vi "2.2.vi"() -> ()   [LabVIEW 2020]
panel:
  out "Valor\nMinimo":dbl
  out "Valor\nMaximo":dbl
  out "Resultados":dbl[][](array[numeric])
  out "Grafica":dbl[](graph)
  # "Grados \nCelsius"
  # "Fahrenheit"
  # "EMA"
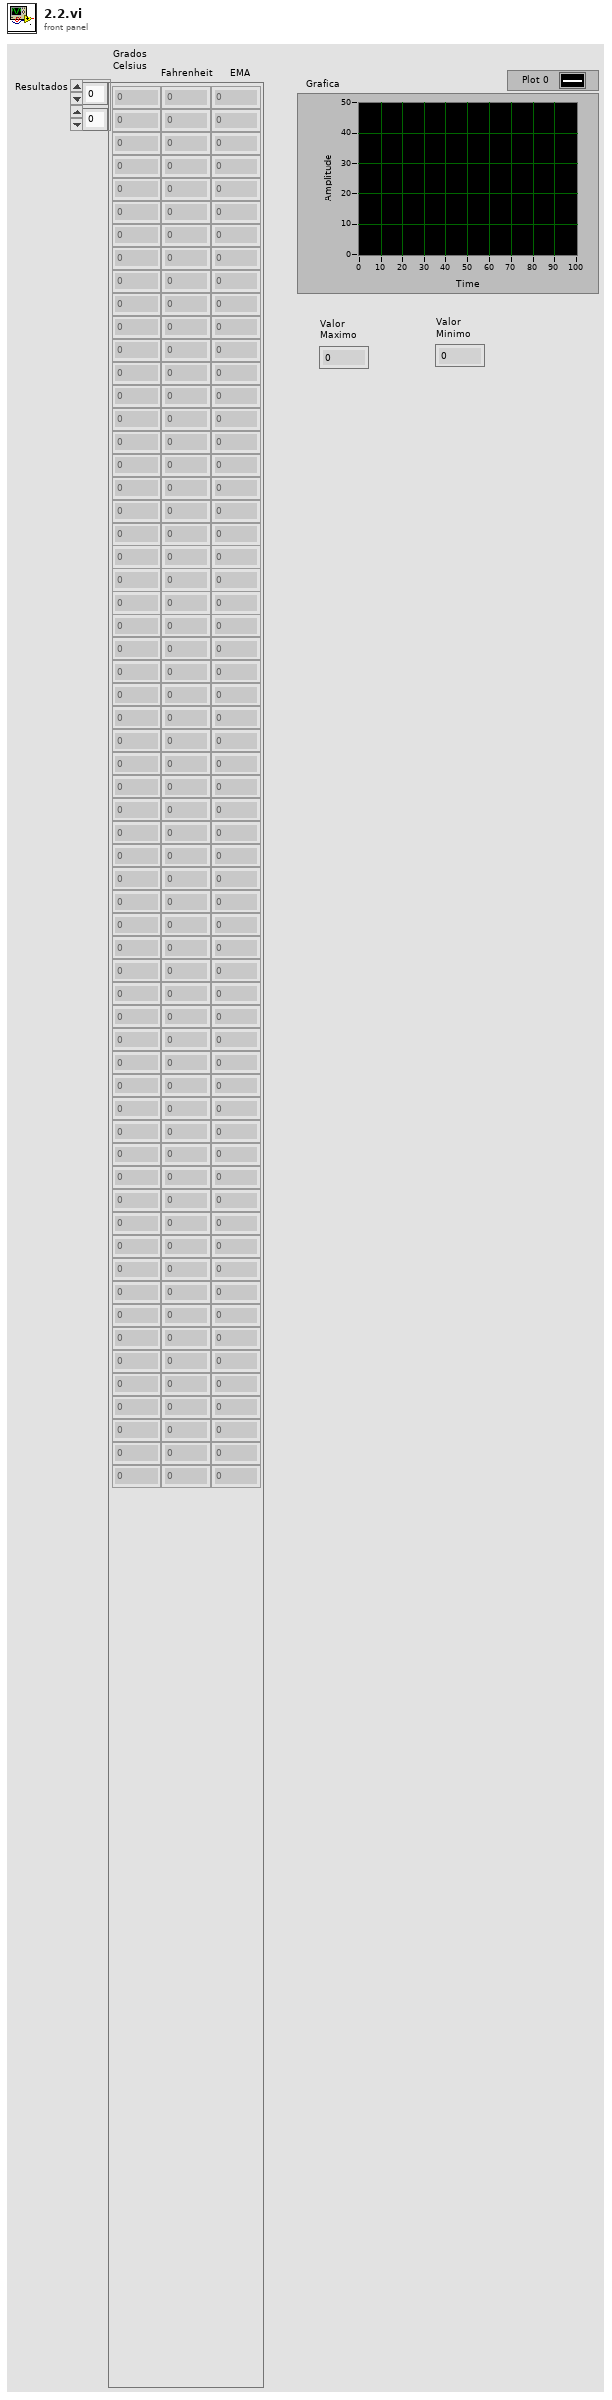
[diagram p1: front panel]
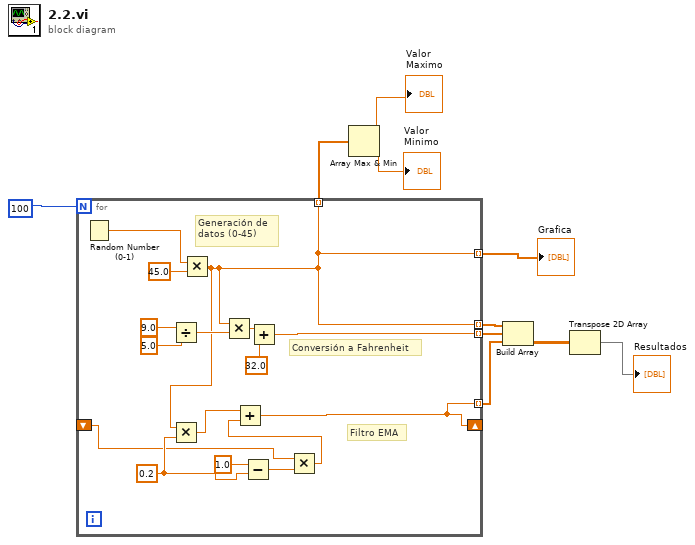
[diagram p0: block diagram]
diagram:
  n1 = for {
    N: 100 -> [_]
    tunnel: [w13] -> w7 mode=indexing
    tunnel: [w19] -> w2 mode=indexing
    tunnel: [w13] -> w6 mode=indexing
    tunnel: [w13] -> w5 mode=indexing
    shift-right: [w11] -> _
    shift-left: _ -> [w12]
    tunnel: [w11] -> w1 mode=indexing
    w15 = 0.2 ("y")
    # "Filtro EMA"
    # "Conversión a Fahrenheit"
    # "Generación de \ndatos (0-45)"
    n2 = Random Number (0-1)() -> (number: 0 to 1=w26:dbl)
    n3 = Divide(x=9.0, y=5.0) -> (x/y=w24:dbl)
    n4 = Multiply(x=w26, y=45.0) -> (x*y=w13:dbl)
    n5 = Multiply(x=w13, y=w15) -> (x*y=w18:dbl)
    n6 = Multiply(x=w13, y=w24) -> (x*y=w21:dbl)
    n7 = Subtract(x=1.0, y=w15) -> (x-y=w16:dbl)
    n8 = Add(x=w21, y=32.0) -> (x+y=w19:dbl)
    n9 = Multiply(x=w12, y=w16) -> (x*y=w17:dbl)
    n10 = Add(x=w18, y=w17) -> (x+y=w11:dbl)
  }
  "Grafica" <- w6
  n11 = Array Max & Min(array=w5) -> (max value=→"Valor\nMaximo":dbl, min value=→"Valor\nMinimo":dbl)  [unwired: 2 out]
  n12 = Build Array(w7, w2, w1) -> (w9:dbl[][])
  n13 = Transpose 2D Array(2D array=w9) -> (transposed array=→"Resultados":dbl[][])
